vi "Flatten.vi"(6 "FIFO Timestamps":T1, 8 "error in (no error)":errorcluster, 10 "Data":T2[](array[typedef]), 11 "CIFTag in":refnum<class "CIF_NIChn_Fifo_Power.lvclass">) -> (0 "error out":errorcluster, 2 "Data out":T2[](array[typedef]), 3 "CIFTag out":refnum<class "CIF_NIChn_Fifo_Power.lvclass">)   [LabVIEW 2021, in "CIF_NIChn_Fifo_Power.lvclass"]
uses:
  CIF_NIChn_Fifo_Power.lvclass
  ChannelCommon/typedef/Datatype Waveform.ctl
  ChannelCommon/typedef/TimeStamps.ctl
  CIF_NIChn_Fifo_Power.lvclass/CIF_NIChn_Fifo_Power.ctl
  ChannelCommon/CIFFIFO/CIFfifo.lvclass/CIFfifo.ctl
  ChannelCommon/CIFFIFO/Accessors/Write T0.vi
  ChannelCommon/CIFFIFO/Accessors/Write T_Out.vi
  <vilib>/CIF Foundation/CIF Utilities/Time/System Time/Get System Time.vi
  ChannelCommon/Utilities/Flatten Header.vi
  ChannelCommon/CIFFIFO/Flatten/Waveform Flatten.vi/6fdbece9-bad6-4a8e-9bf7-fe1528478dd6.vi
  ChannelCommon/CIFFIFO/Flatten/Waveform Flatten.vi/d5e54e4f-7f1a-40ef-960c-6b2cd585230c.vi
  ChannelCommon/CIFFIFO/Flatten/Waveform Flatten.vi/a071385d-aa0c-48d2-a5ce-3b08816305e6.vi
  ChannelCommon/CIFFIFO/Accessors/Write Payload Length.vi
  ChannelCommon/CIFFIFO/Accessors/Read Header.vi
  <vilib>/CIF Foundation/CIF Utilities/Time/System Time/LabVIEW Time to TAI Time.vi
  CIFCore/Common/Utilities/Add Error.vi
  ChannelCommon/CIFFIFO/Flatten/Waveform Flatten.vi/6fdbece9-bad6-4a8e-9bf7-fe1528478dd6.vi/c28b0ead-42ad-4072-80a2-aca7f2bd7ce3.vi
  ChannelCommon/CIFFIFO/Flatten/Waveform Flatten.vi/d5e54e4f-7f1a-40ef-960c-6b2cd585230c.vi/c28b0ead-42ad-4072-80a2-aca7f2bd7ce3.vi
  ChannelCommon/CIFFIFO/Flatten/Waveform Flatten.vi/a071385d-aa0c-48d2-a5ce-3b08816305e6.vi/c28b0ead-42ad-4072-80a2-aca7f2bd7ce3.vi
  <vilib>/CIF Foundation/CIF Utilities/Errors/Append Error Location.vi
  ChannelCommon/CIFFIFO/CIFfifo.lvclass
  ChannelCommon/ChannelCommon.lvlib
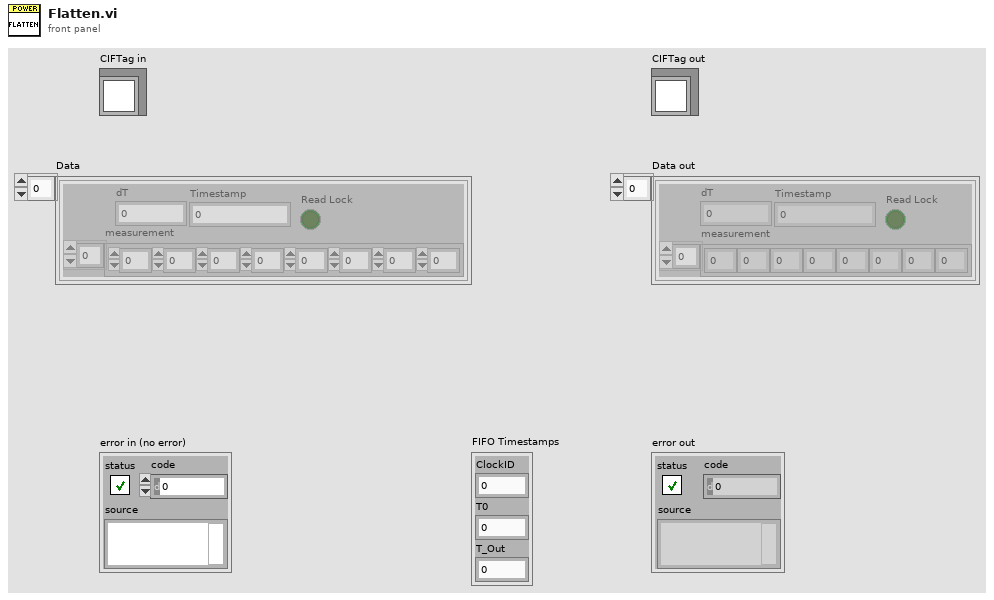
[diagram p1: front panel]
types:
  T1 = typedef "ChannelCommon.lvlib/TimeStamps.ctl" = cluster{"ClockID":u8, "T0":i64, "T_Out":i64}
  T2 = typedef "ChannelCommon.lvlib/Datatype Waveform.ctl" = cluster{"measurement":dbl[], "dT":dbl, "Timestamp":u64, "Read Lock":bool}
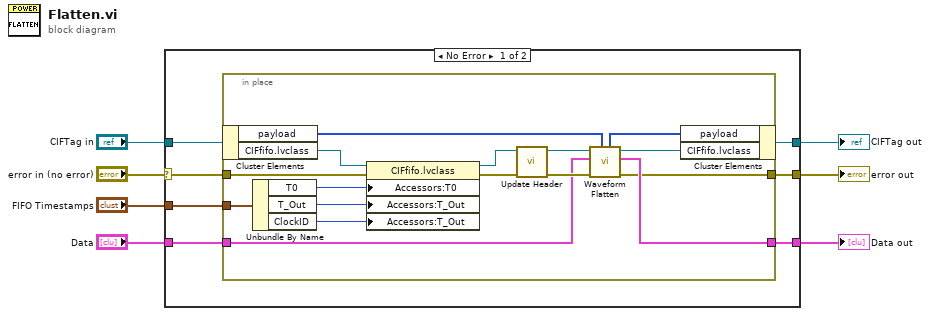
[diagram p0: block diagram]
diagram:
  n1 = case shown="No Error" "error in (no error)" {
    selector: "error in (no error)" -> [w9 w33]
    tunnel: [w14 w33] -> w6
    tunnel: [w13 w32] -> w4
    tunnel: "CIFTag in" -> [w10 w32]
    tunnel: "Data" -> [w12 w31]
    tunnel: [w11 w31] -> w2
    tunnel: "FIFO Timestamps" -> [w8 _]
    frame No Error {
      n2 = in-place {
        in-place-border: w9 -> [w27]
        in-place-border: [w19] -> w14
        in-place-border: w12 -> [w23]
        in-place-border: [w20] -> w11
        in-place-border: w8 -> [w18]
        n3 = in-place-cluster #1(w10) -> ("payload"=w24:u8[], "CIFfifo.lvclass"=w30:refnum<class "CIFfifo.lvclass">)
        n4 = Unbundle By Name(w18) -> ("T0"=w17:i64, "T_Out"=w16:i64, "ClockID"=w15:u8)
        n5 = property class="CIFfifo.lvclass"(reference=w30, error in=w27, "Accessors:T0"=w17, "Accessors:T_Out"=w16, "Accessors:T_Out"=w15) -> (reference out=w29:refnum<class "CIFfifo.lvclass">, error out=w28:errorcluster)
        n6 = call "Update Header.vi"("error in (no error)"=w28, "CIFFIFO in"=w29) -> ("error out"=w25:errorcluster, "CIFFIFO out"=w26:refnum<class "CIFfifo.lvclass">)  [unwired: 8 in]
        n7 = call "Waveform Flatten.vi"("payload in"=w24, "error in (no error)"=w25, "Data in"=w23, "CIFFifo in"=w26) -> ("error out"=w19:errorcluster, "Data out"=w20:T2[], "CIFFifo out"=w21:refnum<class "CIFfifo.lvclass">, "payload out"=w22:u8[])  [unwired: 3 in, 1 out]
        n8 = in-place-cluster #1("payload"=w22, "CIFfifo.lvclass"=w21) -> (w13:refnum<class "CIF_NIChn_Fifo_Power.lvclass">)
      }
    }
    frame Error {
    }
  }
  "error out" <- w6
  "CIFTag out" <- w4
  "Data out" <- w2
